vi "Stop.vi"(8 "Error In":errorcluster, 11 "AutoData":T1) -> (0 "Error Out":errorcluster, 3 "AutoData out":T1)   [LabVIEW 2019, in "AutoMode.lvlib"]
uses:
  AutoMode.lvlib
  Cluster - AutoModeData.ctl
  MainController/Cluster - TestSettings.ctl
  MainController/Cluster - HardwareConfiguration.ctl
  MainController/Cluster - TestResults.ctl
  Cluster - AutoModeMessage.ctl
  Enum - AutoModeState.ctl
  MainController/Cluster - MainControllerMessage.ctl
  MainController/Enum - MainState.ctl
  Mark10 API/WriteStopMove.vi
  MainController/MainController.lvlib
  Mark10 API/Mark 10 TSTM-DC.lvlib
  EventLogger/EventLogger.lvlib
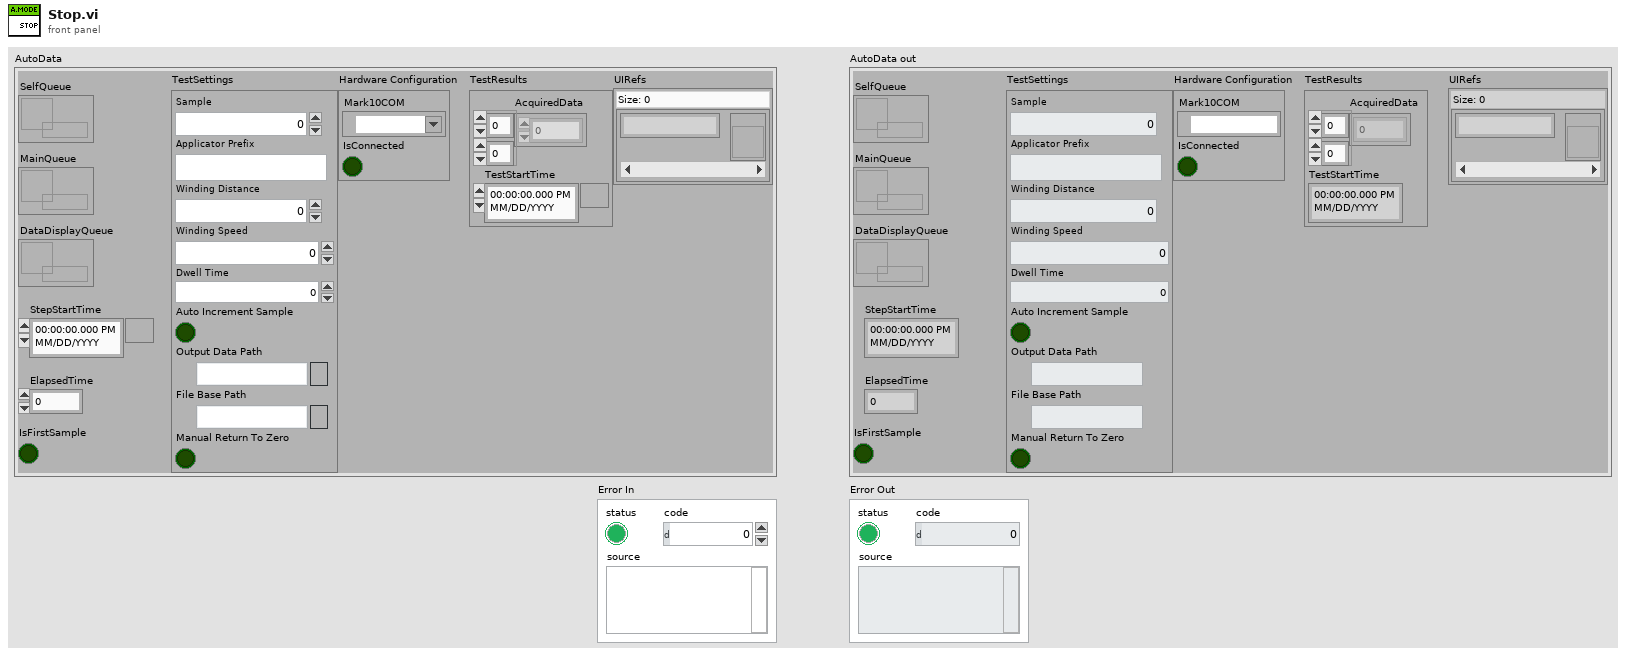
[diagram p1: front panel]
types:
  T1 = typedef "AutoMode.lvlib/Cluster - AutoModeData.ctl" = cluster{"DataDisplayQueue":refnum<queue>, "StepStartTime":timestamp, "TestSettings":T2, "Hardware Configuration":T3, "TestResults":T4, "ElapsedTime":dbl, "IsFirstSample":bool, "UIRefs":map{string, refnum<vi>}, "SelfQueue":refnum<queue>, "MainQueue":refnum<queue>}
  T2 = typedef "MainController.lvlib/Cluster - TestSettings.ctl" = cluster{"Sample":u32, "Applicator Prefix":string, "Winding Distance":dbl, "Winding Speed":dbl, "Dwell Time":dbl, "Auto Increment Sample":bool, "Output Data Path":path, "File Base Path":path, "Manual Return To Zero":bool}
  T3 = typedef "MainController.lvlib/Cluster - HardwareConfiguration.ctl" = cluster{"Mark10COM":refnum<visa-resource-name>, "IsConnected":bool}
  T4 = typedef "MainController.lvlib/Cluster - TestResults.ctl" = cluster{"AcquiredData":dbl[][], "TestStartTime":timestamp}
  T5 = typedef "MainController.lvlib/Enum - MainState.ctl" = enum16{"Initialize", "InitUIRefs", "LaunchSettings", "LaunchAutoMode", "LaunchManualMode", "LaunchTestReport", "ConnectHardware", "DisconnectHardware", "HiliteNavItems", "StartAutoMode", "PauseAutoMode", "StopAutoMode", "ShowFlyout", "HideFlyout", "BroadcastSettings", "PickupTestSettings", "BroadcastHW", "AutoTestDone", "DAQStatus", "UpdateCommandBar", "Error", "RecieveError", "Exit"}
  T6 = typedef "AutoMode.lvlib/Enum - AutoModeState.ctl" = enum16{"Initialize", "Idle", "UpdateConfig", "UpdateHWConfig", "BroadcastSettings", "Start", "CheckValidReportPath", "Winding", "WaitForWinding", "Unwind", "WaitForUnwind", "Stop", "Abort", "WriteDataToFile", "EventTriggered", "GenerateFilePath", "ZeroPosition", "GotoZero", "Error", "Exit"}
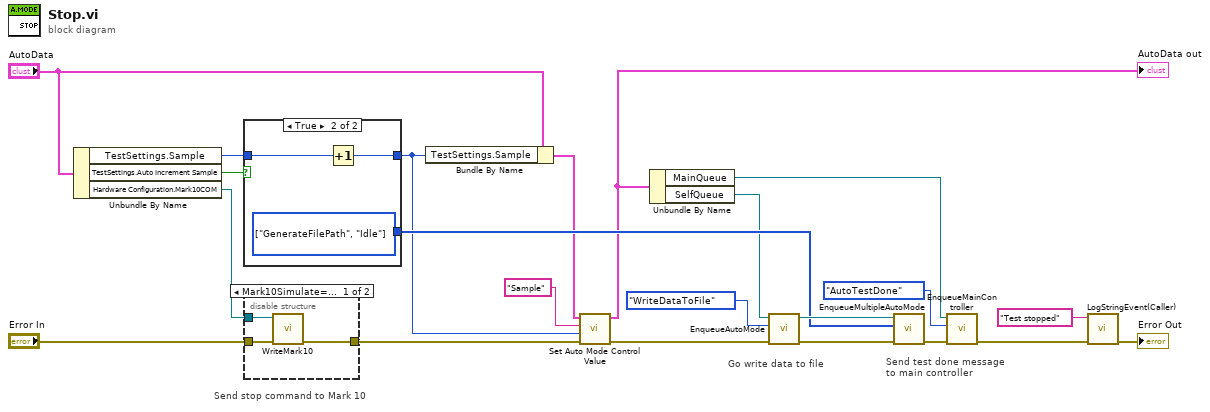
[diagram p0: block diagram]
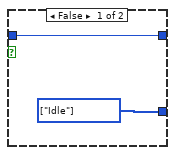
[diagram p2: hidden frame]
diagram:
  # "Send test done message to main controller"
  # "Go write data to file"
  # "Send stop command to Mark 10"
  n1 = Unbundle By Name("AutoData") -> ("TestSettings.Sample"=w14:u32, "TestSettings.Auto Increment Sample"=w15:bool, "Hardware Configuration.Mark10COM"=w21:refnum<visa-resource-name>)
  n2 = case shown="True" w15 {
    tunnel: w14 -> [w24 w27]
    tunnel: [w24 w26] -> w3
    tunnel: [w23 w25] -> w13
    frame False {
      w23 = T6[] [enum."Idle"] items=["Initialize", "Idle", "UpdateConfig", "UpdateHWConfig", "BroadcastSettings", "Start", "CheckValidReportPath", "Winding", "WaitForWinding", "Unwind", "WaitForUnwind", "Stop", "Abort", "WriteDataToFile", "EventTriggered", "GenerateFilePath", "ZeroPosition", "GotoZero", "Error", "Exit"] ("CycleTestState")
    }
    frame True {
      w25 = T6[] [enum."GenerateFilePath", enum."Idle"] items=["Initialize", "Idle", "UpdateConfig", "UpdateHWConfig", "BroadcastSettings", "Start", "CheckValidReportPath", "Winding", "WaitForWinding", "Unwind", "WaitForUnwind", "Stop", "Abort", "WriteDataToFile", "EventTriggered", "GenerateFilePath", "ZeroPosition", "GotoZero", "Error", "Exit"] ("CycleTestState")
      n3 = Increment(x=w27) -> (x+1=w26:u32)
    }
  }
  n4 = disable-structure shown="Mark10Simulate==False, Default" {
    disable-tunnel: "Error In" -> [w30 w31]
    disable-tunnel: [w29 w31] -> w22
    disable-tunnel: w21 -> [w28 _]
    frame condition #0 (active) {
      n5 = call-poly "WriteMark10.vi"("error in"=w30, "VISA resource name"=w28) -> ("error out"=w29:errorcluster)  [unwired: 8 in, 1 out]
    }
    frame condition #1 {
    }
  }
  n6 = Bundle By Name(cluster="AutoData", "TestSettings.Sample"=w3) -> (w6:T1)
  n7 = call "Set Auto Mode Control Value.vi"("Error In"=w22, "Value"=w3, "key"="Sample", "AutoData"=w6) -> ("Error Out"=w7:errorcluster, "AutoData out"=w5:T1)  [unwired: 6 in]
  "AutoData out" <- w5
  n8 = Unbundle By Name(w5) -> ("MainQueue"=w12:refnum<queue>, "SelfQueue"=w8:refnum<queue>)
  n9 = call "EnqueueAutoMode.vi"("error in (no error)"=w7, "AutoState"=Enum_-_AutoModeState."WriteDataToFile" ("CycleTestState"), "Queue in"=w8) -> ("error out"=w18:errorcluster, "queue out"=w19:refnum<queue>)  [unwired: 7 in]
  n10 = call "EnqueueMultipleAutoMode.vi"("error in (no error)"=w18, "AutoState"=w13, "Queue in"=w19) -> ("error out"=w16:errorcluster)  [unwired: 7 in, 1 out]
  n11 = call "EnqueueMainController.vi"("error in (no error)"=w16, "Message"=Enum_-_MainState."AutoTestDone", "MainQueue"=w12) -> ("error out"=w10:errorcluster)  [unwired: 6 in, 2 out]
  n12 = call "LogStringEvent(Caller).vi"("Error In"=w10, "Field"="Test stopped") -> ("Error Out"=→"Error Out":errorcluster)  [unwired: 9 in]
